vi "Add Two Inputs.vi"(1 "in 2":sgl, 9 "in 1":sgl) -> (7 "Numeric":sgl)   [LabVIEW 2014]
doc: "Simple add but has inputs on sides and output on top."
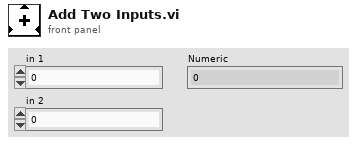
[diagram p1: front panel]
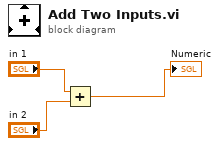
[diagram p0: block diagram]
diagram:
  n1 = Add(x="in 1", y="in 2") -> (x+y=→"Numeric":sgl)
